vi "Create Active Axis Name.vi"(8 "error in (no error)":errorcluster, 10 "Alignment Lens":enum16{"Collimator", "FAC", "SAC"}(ring), 11 "Newport in":refnum<class "Newport.lvclass">) -> (0 "error out":errorcluster, 2 "Alignment Axis":string, 3 "Newport out":refnum<class "Newport.lvclass">)   [LabVIEW 2018, in "Newport.lvlib" / "Newport.lvclass"]
uses:
  Newport.lvclass
  C:/Projects/LabVIEW/In-Progress/Chetan Malpure/Axis/Parent/Axis.lvclass
  Parent/Axis.lvclass/Axis.ctl
  Parent/Axis.lvclass
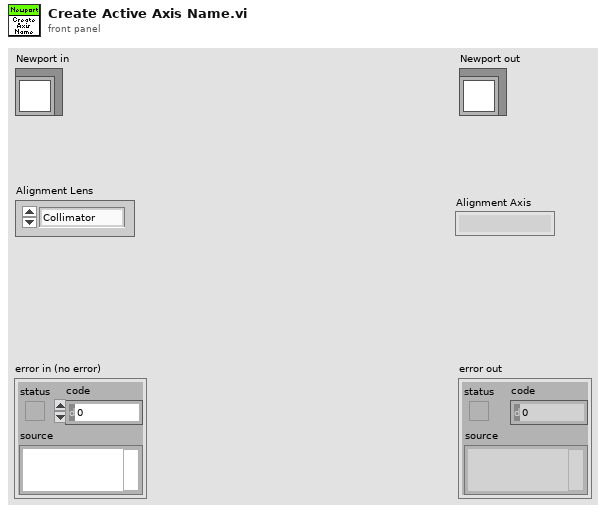
[diagram p1: front panel]
types:
  T1 = typedef "Axis.lvlib/Axis.ctl" = enum16{"None", "X", "Y", "Z", "Rx", "Ry", "Rz"}
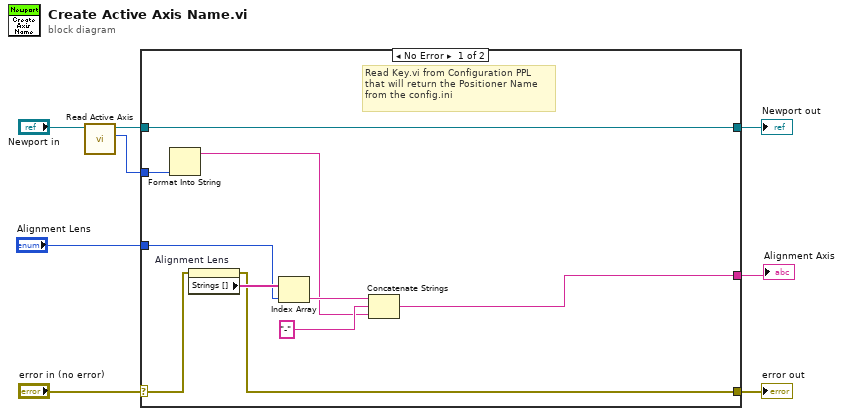
[diagram p0: block diagram]
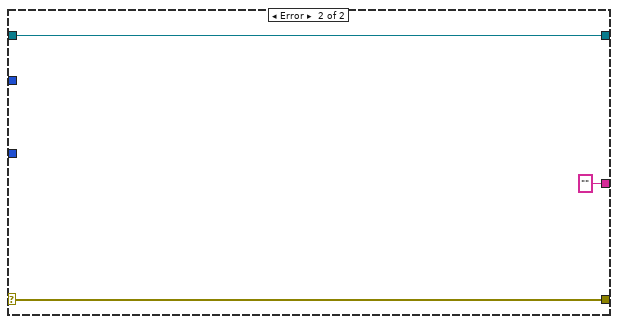
[diagram p2: hidden frame]
diagram:
  n1 = call "Read Active Axis.vi"("Axis in"="Newport in") -> ("Axis"=w3:T1, "Axis out"=w4:refnum<class "Newport.lvclass">)  [unwired: 8 in, 1 out]
  n2 = case shown="No Error" "error in (no error)" {
    selector: "error in (no error)" -> [w10 w21]
    tunnel: [w9 w21] -> w7
    tunnel: [w18 w20] -> w6
    tunnel: w4 -> [w18 w20]
    tunnel: w3 -> [w15 _]
    tunnel: "Alignment Lens" -> [w16 _]
    tunnel: [w11 ""] -> w1
    frame No Error {
      # "Read Key.vi from Configuration PPL\nthat will return the Positioner Name\nfrom the config.ini"
      n3 = Format Into String(w15) -> (resulting string=w12:string)  [unwired: 3 in, 1 out]
      n4 = property on="Alignment Lens" class="Enum (strict)"(error in=w10) -> (error out=w9:errorcluster, "Strings []"=w17:string[])  [unwired: 1 in, 1 out]
      n5 = Index Array(array=w17, index=w16) -> (element=w14:string)
      n6 = Concatenate Strings(w14, "-" ("string"), w12) -> (w11:string)
    }
    frame Error {
    }
  }
  "error out" <- w7
  "Newport out" <- w6
  "Alignment Axis" <- w1
